vi "Panel.vi"(11 "CheckboxControlEditorPanel in":refnum<class "CheckboxControlEditorPanel.lvclass">) -> ()   [LabVIEW 2020, in "VolatusGUIControls.lvlib" / "CheckboxControlEditorPanel.lvclass"]
uses:
  CheckboxControlEditorPanel.lvclass
  C:/dev/lv20CE/relink/volatus-gui-controls/VolatusGUIEditorCore/ElementEditorPanel/ElementEditorPanel.lvclass
  C:/dev/lv20CE/relink/lv-oopanel/OOPanel/Panel/Panel.lvclass
  lv-oopanel/OOPanel/Panel/Basic UI State.ctl
  lv-autocomplete/AutoComplete/AutoComplete/AutoComplete.lvclass/AutoComplete.ctl
  CheckboxControlEditorPanel.lvclass/CheckboxControlEditorPanel.ctl
  lv-autocomplete/AutoComplete/Launch Autocomplete Handler.vi
  lv-autocomplete/AutoComplete/AutoComplete/AutoComplete.lvclass
  lv-oopanel/OOPanel/Panel/Panel.lvclass
  lv-oopanel/OOPanel/OOPanel.lvlib
  VolatusGUIEditorCore/ElementEditorPanel/ElementEditorPanel.lvclass
  VolatusGUIEditorCore/VolatusGUIEditorCore.lvlib
panel:
  in  "Top":i32
  in  "Left":i32
  in  "Height":u16
  in  "Width":u16
  in  "Label Text Color":u32(colorbox) caption="Color"
  in  "Label Visible":bool caption="Visible"
  in  "Label":string
  in  "Channel":string
  in  "True Color":u32(colorbox)
  in  "False Color":u32(colorbox)
  # "Label"
  # "False"
  # "True"
  # "Color"
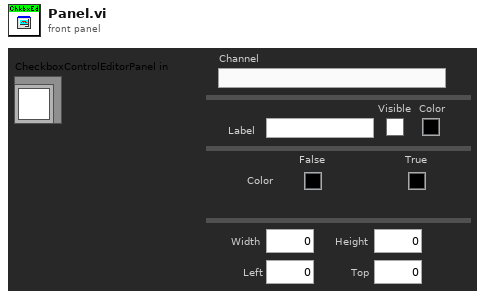
[diagram p1: front panel]
types:
  T1 = typedef "OOPanel.lvlib/Panel.lvclass/Basic UI State.ctl" = enum16{"Init", "Run", "Close"}
  T2 = typedef "VolatusGUIEditorCore.lvlib/ElementEditorPanel.lvclass/Incoming Events.ctl" = cluster{"Update Control":refnum<user-event>}
  T3 = typedef "OOPanel.lvlib/Panel.lvclass/Panel Events.ctl" = cluster{"Visbility":refnum<user-event>, "Close":refnum<user-event>}
  T4 = typedef "VolatusGUIControls.lvlib/CheckboxControlEditorPanel.lvclass/Props.ctl" = cluster{"JSON":T5, "Label":T6, "Position":T7, "Width":u16, "Height":u16, "Boolean Colors":T8}
  T5 = typedef "VolatusGUIControls.lvlib/CheckboxControlEditorPanel.lvclass/JSON Props.ctl" = cluster{"Channel":string}
  T6 = typedef "VolatusGUIEditorCore.lvlib/Label Props.ctl" = cluster{"Text":string, "Text Color":u32, "Visible":bool}
  T7 = typedef "VolatusGUIEditorCore.lvlib/Position Props.ctl" = cluster{"Left":i32, "Top":i32}
  T8 = typedef "VolatusGUIEditorCore.lvlib/Boolean Color Props.ctl" = cluster{"False":u32, "True":u32}
  T9 = typedef "OOPanel.lvlib/Visibility State.ctl" = enum16{"Idle", "Closed", "Hidden", "Visible", "Subpanel", "Hidden Subpanel"}
  T10 = cluster{"Label":string, "Label Text Color":u32, "Label Visible":bool}
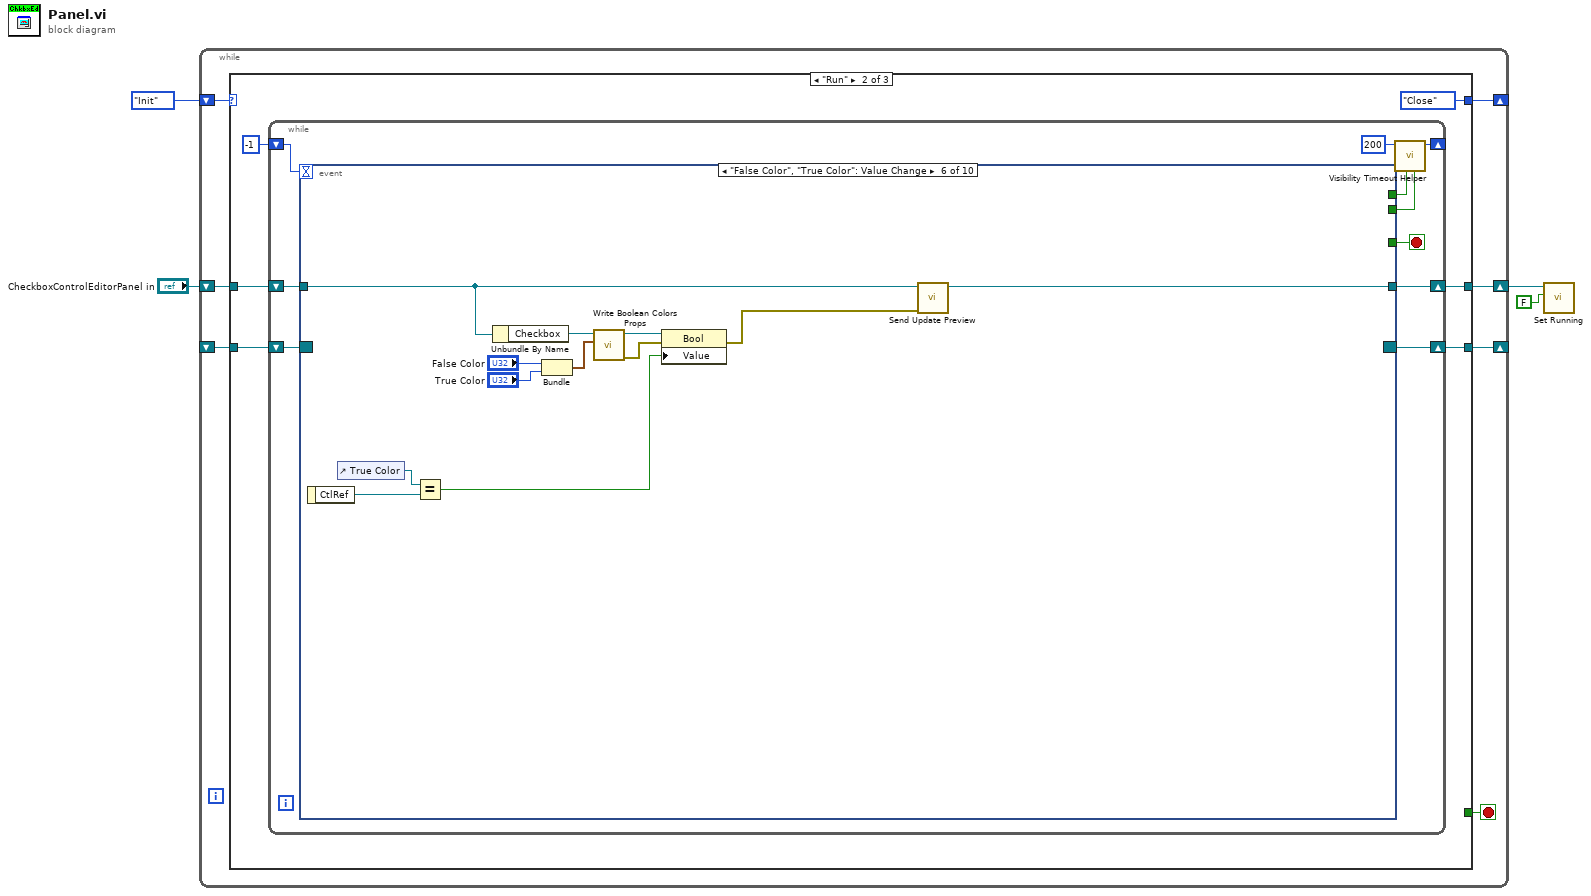
[diagram p0: block diagram]
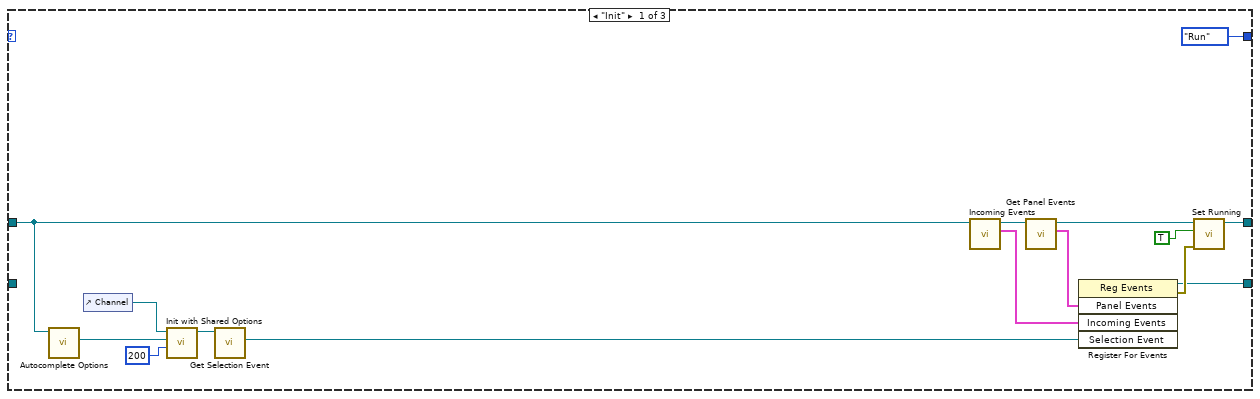
[diagram p2: hidden frame]
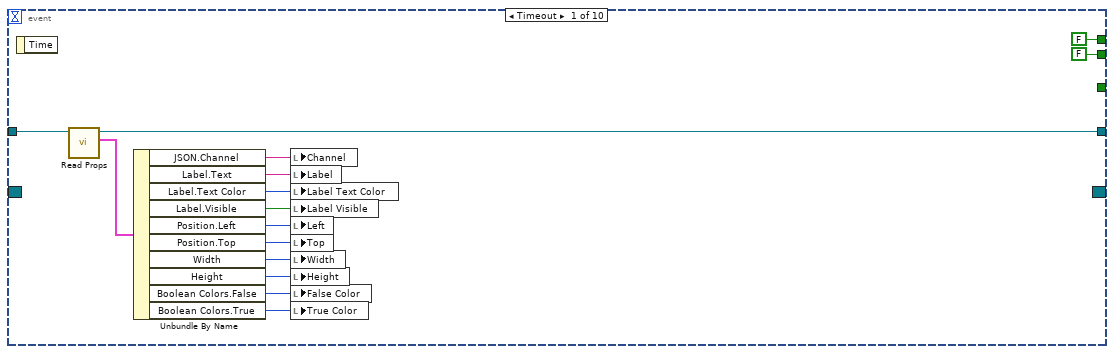
[diagram p3: hidden frame]
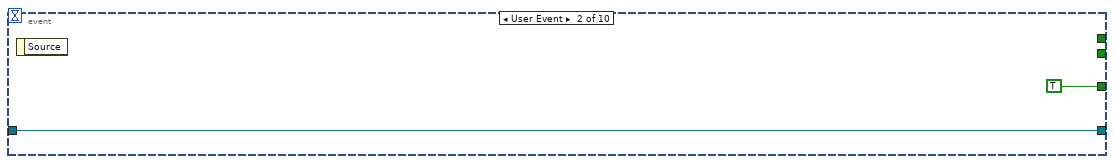
[diagram p4: hidden frame]
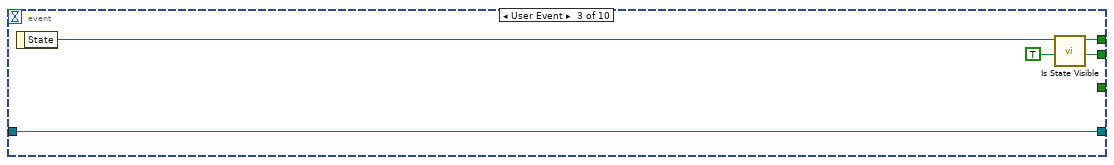
[diagram p5: hidden frame]
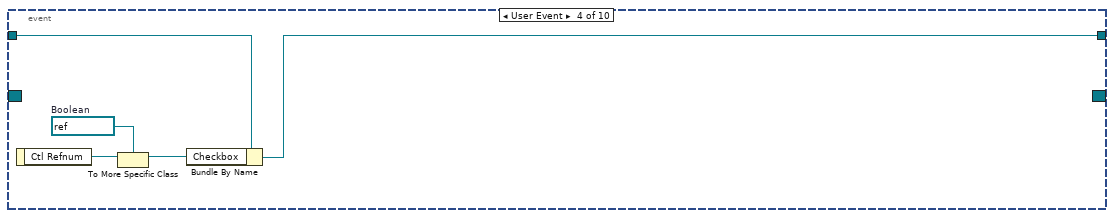
[diagram p6: hidden frame]
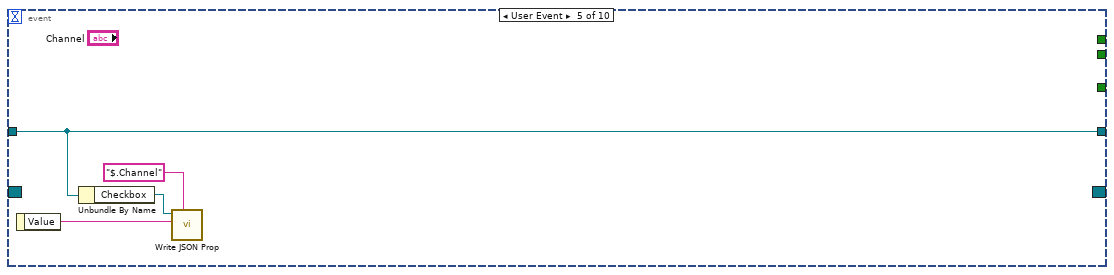
[diagram p7: hidden frame]
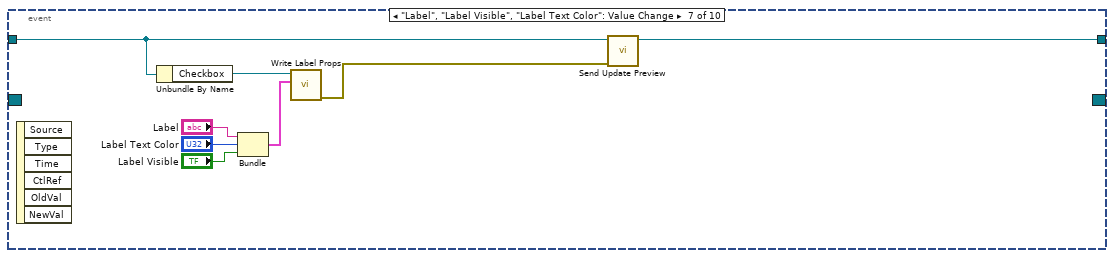
[diagram p8: hidden frame]
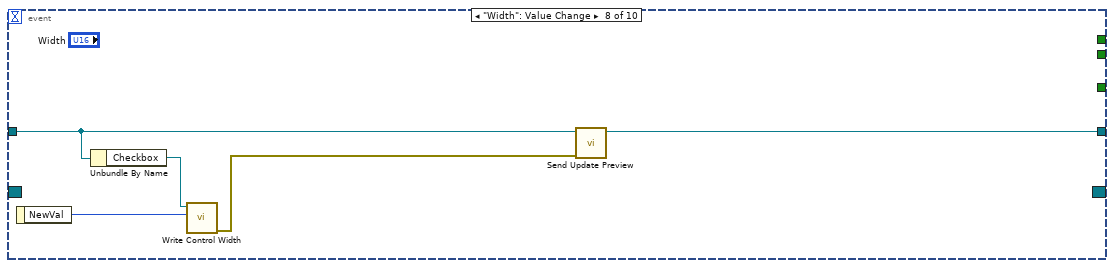
[diagram p9: hidden frame]
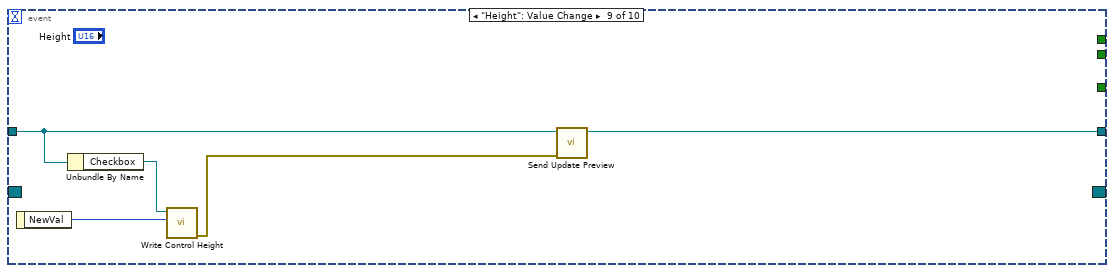
[diagram p10: hidden frame]
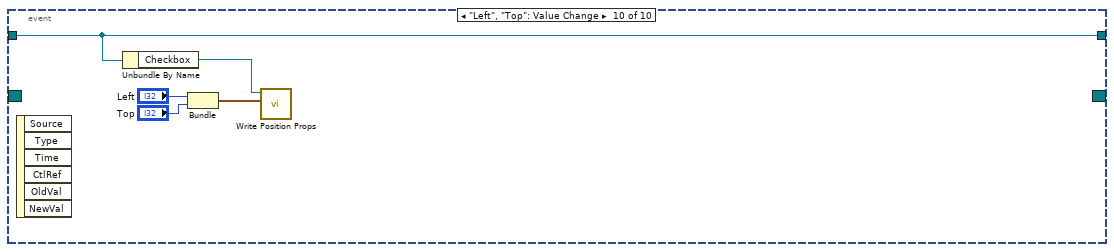
[diagram p11: hidden frame]
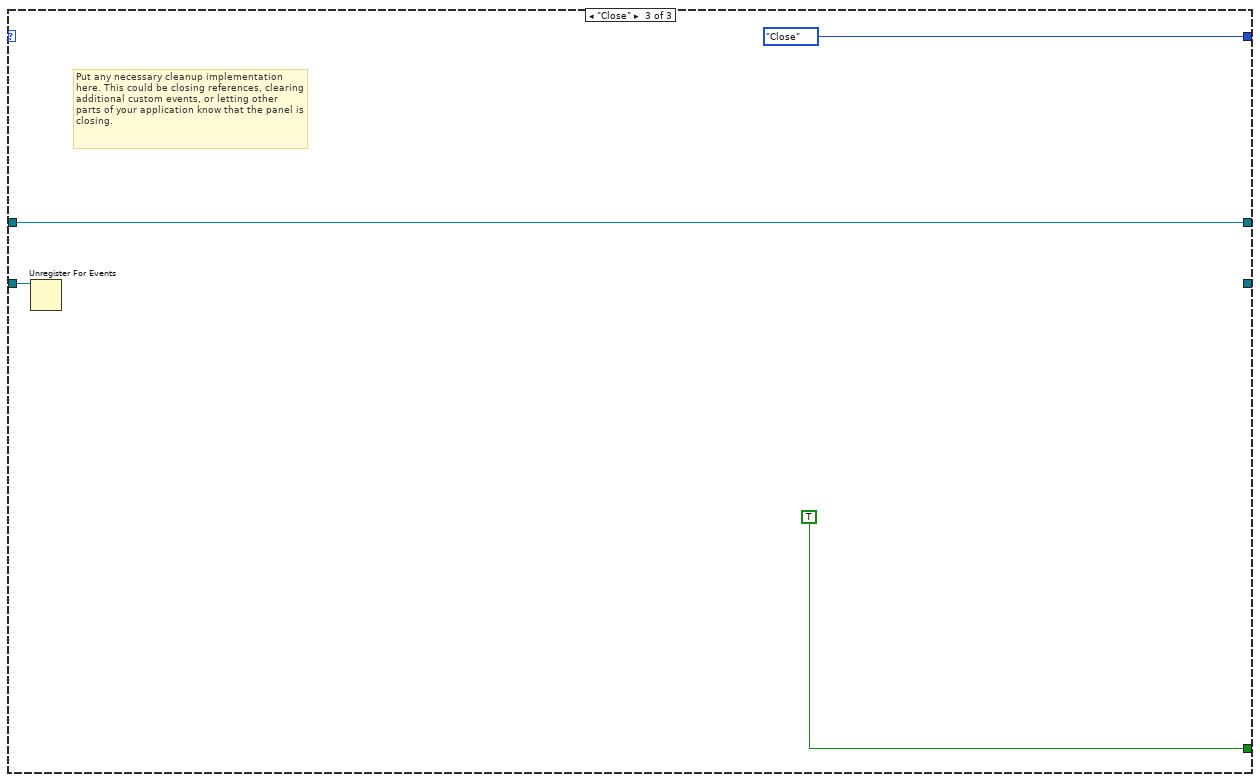
[diagram p12: hidden frame]
diagram:
  n1 = while {
    shift-right: [w10] -> _
    shift-left: _ -> [w11]
    shift-right: [w8] -> _
    shift-left: Basic_UI_State."Init" ("Basic UI State") -> [w9]
    shift-right: [w6] -> w4
    shift-left: "CheckboxControlEditorPanel in" -> [w5]
    stop <- w7 stop-if-true
    n2 = case shown="\"Run\"" w9 {
      tunnel: w11 -> [_ w32 w109]
      tunnel: [w23 w30 _] -> w10
      tunnel: [Basic_UI_State."Run" ("Basic UI State") Basic_UI_State."Close" ("Basic UI State") Basic_UI_State."Close" ("Basic UI State")] -> w8
      tunnel: [_ _ TRUE] -> w7
      tunnel: [w22 w27 w108] -> w6
      tunnel: w5 -> [w14 w28 w108]
      frame "Init" {
        n3 = call "Autocomplete Options.vi"("ElementEditorPanel in"=w14) -> ("Autocomplete Options"=w17:refnum<class "Shared Options.lvclass">)  [unwired: 10 in]
        n4 = control-ref of="Channel"() -> (w12:refnum<vi>)
        n5 = call "Init with Shared Options.vi"("Height (200)"=i16 200, "Shared Options"=w17, "Str Refnum"=w12) -> ("AutoComplete out"=w16:refnum<class "AutoComplete.lvclass">)  [unwired: 7 in, 1 out]
        n6 = call "Get Selection Event.vi"("AutoComplete in"=w16) -> ("Selection Event"=w13:refnum<user-event>)  [unwired: 9 in, 1 out]
        n7 = call "Incoming Events.vi"("ElementEditorPanel in"=w14) -> ("Incoming Events"=w18:T2, "ElementEditorPanel out"=w19:refnum<class "CheckboxControlEditorPanel.lvclass">)  [unwired: 9 in]
        n8 = call "Get Panel Events.vi"("Panel in"=w19) -> ("Panel Events"=w20:T3, "Panel out"=w21:refnum<class "CheckboxControlEditorPanel.lvclass">)  [unwired: 8 in, 1 out]
        n9 = register-events(w20, w18, w13) -> (reference out=w23:refnum<event-registration>, error out=w25:errorcluster)  [unwired: 2 in]
        n10 = call "Set Running.vi"("error in (no error)"=w25, "Running"=TRUE, "Panel in"=w21) -> ("Panel out"=w22:refnum<class "CheckboxControlEditorPanel.lvclass">)  [unwired: 7 in, 1 out]
      }
      frame "Run" {
        n11 = while {
          shift-right: [w38] -> w30
          shift-left: w32 -> [w39]
          shift-right: [w41] -> _
          shift-left: -1 ("Timeout") -> [w40]
          shift-right: [w33] -> w27
          shift-left: w28 -> [w34]
          stop <- w35 stop-if-true
          n12 = event shown="[5] \"False Color\", \"True Color\": Value Change" {
            selector: w39 -> [_ _ _ _ _ _ _ _ _ _]
            dyn-events: [_ _ _ _ _ _ _ _ _ _] -> w38
            timeout: w40 -> [_ _ _ _ _ _ _ _ _ _]
            tunnel: [FALSE _ w62 _ _ _ _ _ _ _] -> w37
            tunnel: [FALSE _ TRUE _ _ _ _ _ _ _] -> w36
            tunnel: [_ TRUE _ _ _ _ _ _ _ _] -> w35
            tunnel: w34 -> [w54 w58 w60 w68 w70 w81 w88 w97 w102 w105]
            tunnel: [w55 w58 w60 w65 w70 w79 w86 w94 w99 w105] -> w33
            event Timeout {
              n13 = event-data() -> ()  [unwired: 1 in, 1 out]
              n14 = call "Read Props.vi"("CheckboxControlEditorPanel in"=w54) -> ("Props"=w53:T4, "CheckboxControlEditorPanel out"=w55:refnum<class "CheckboxControlEditorPanel.lvclass">)  [unwired: 8 in, 1 out]
              n15 = Unbundle By Name(w53) -> ("JSON.Channel"=w52:string, "Label.Text"=w43:string, "Label.Text Color"=w51:u32, "Label.Visible"=w50:bool, "Position.Left"=w49:i32, "Position.Top"=w48:i32, "Width"=w47:u16, "Height"=w46:u16, "Boolean Colors.False"=w45:u32, "Boolean Colors.True"=w44:u32)
              n16 = local write "Channel"(w52) -> ()
              n17 = local write "Label"(w43) -> ()
              n18 = local write "Label Text Color"(w51) -> ()
              n19 = local write "Label Visible"(w50) -> ()
              n20 = local write "Left"(w49) -> ()
              n21 = local write "Top"(w48) -> ()
              n22 = local write "Width"(w47) -> ()
              n23 = local write "Height"(w46) -> ()
              n24 = local write "False Color"(w45) -> ()
              n25 = local write "True Color"(w44) -> ()
            }
            event User Event {
              n26 = event-data() -> ()  [unwired: 1 in, 1 out]
            }
            event User Event {
              n27 = event-data() -> ("State"=w63:T9)  [unwired: 1 in]
              n28 = call "Is State Visible.vi"("Visibility"=w63) -> ("Visible"=w62:bool)  [unwired: 10 in]
            }
            event User Event {
              w66 = refnum<vi> refnum  # Boolean
              n29 = event-data() -> ("Ctl Refnum"=w67:refnum<vi>)  [unwired: 1 in]
              n30 = To More Specific Class(target class=w66, reference=w67) -> (specific class reference=w64:refnum<vi>)  [unwired: 1 in, 1 out]
              n31 = Bundle By Name(cluster=w68, "Checkbox"=w64) -> (w65:refnum<class "CheckboxControlEditorPanel.lvclass">)
            }
            event User Event {
              n32 = event-data() -> ("Value"=w69:string)  [unwired: 1 in]
              n33 = Unbundle By Name(w70) -> ("Checkbox"=w72:refnum<vi>)
              n34 = call "Write JSON Prop.vi"("JSON Path"="$.Channel" ("$Path or Item Name"), "Value"=w69, "Ctl Refnum in"=w72) -> ()  [unwired: 7 in, 2 out]
            }
            event "False Color", "True Color": Value Change {
              n35 = event-data() -> ("CtlRef"=w78:refnum<vi>)  [unwired: 1 in]
              n36 = control-ref of="True Color"() -> (w77:refnum<vi>)
              n37 = Equal?(x=w77, y=w78) -> (x = y?=w74:bool)
              n38 = Unbundle By Name(w81) -> ("Checkbox"=w80:refnum<vi>)
              n39 = Bundle("False Color"="False Color", "True Color"="True Color") -> (w82:cluster{"False Color":u32, "True Color":u32})  [unwired: 1 in]
              n40 = call "Write Boolean Colors Props.vi"("Boolean Colors Props"=w82, "Control in"=w80) -> ("error out"=w75:errorcluster, "Control"=w76:refnum<vi>)  [unwired: 8 in]
              n41 = property class="Bool"(reference=w76, error in=w75, "Value"=w74) -> (error out=w73:errorcluster)  [unwired: 1 out]
              n42 = call "Send Update Preview.vi"("error in (no error)"=w73, "ElementEditorPanel in"=w81) -> ("ElementEditorPanel out"=w79:refnum<class "CheckboxControlEditorPanel.lvclass">)  [unwired: 8 in, 1 out]
            }
            event "Label", "Label Visible", "Label Text Color": Value Change {
              n43 = event-data() -> ()  [unwired: 1 in, 6 out]
              n44 = Unbundle By Name(w88) -> ("Checkbox"=w87:refnum<vi>)
              n45 = Bundle("Label"="Label", "Label Text Color"="Label Text Color", "Label Visible"="Label Visible") -> (w89:T10)  [unwired: 1 in]
              n46 = call "Write Label Props.vi"("Label Props"=w89, "Ctl Refnum in"=w87) -> ("error out"=w85:errorcluster)  [unwired: 8 in, 1 out]
              n47 = call "Send Update Preview.vi"("error in (no error)"=w85, "ElementEditorPanel in"=w88) -> ("ElementEditorPanel out"=w86:refnum<class "CheckboxControlEditorPanel.lvclass">)  [unwired: 8 in, 1 out]
            }
            event "Width": Value Change {
              n48 = event-data() -> ("NewVal"=w95:u16)  [unwired: 1 in]
              n49 = Unbundle By Name(w97) -> ("Checkbox"=w96:refnum<vi>)
              n50 = call "Write Control Width.vi"("Width"=w95, "Control in"=w96) -> ("error out"=w93:errorcluster)  [unwired: 8 in, 1 out]
              n51 = call "Send Update Preview.vi"("error in (no error)"=w93, "ElementEditorPanel in"=w97) -> ("ElementEditorPanel out"=w94:refnum<class "CheckboxControlEditorPanel.lvclass">)  [unwired: 8 in, 1 out]
            }
            event "Height": Value Change {
              n52 = event-data() -> ("NewVal"=w100:u16)  [unwired: 1 in]
              n53 = Unbundle By Name(w102) -> ("Checkbox"=w101:refnum<vi>)
              n54 = call "Write Control Height.vi"("Height"=w100, "Control in"=w101) -> ("error out"=w98:errorcluster)  [unwired: 8 in, 1 out]
              n55 = call "Send Update Preview.vi"("error in (no error)"=w98, "ElementEditorPanel in"=w102) -> ("ElementEditorPanel out"=w99:refnum<class "CheckboxControlEditorPanel.lvclass">)  [unwired: 8 in, 1 out]
            }
            event "Left", "Top": Value Change {
              n56 = event-data() -> ()  [unwired: 1 in, 6 out]
              n57 = Unbundle By Name(w105) -> ("Checkbox"=w104:refnum<vi>)
              n58 = Bundle("Left"="Left", "Top"="Top") -> (w103:cluster{"Left":i32, "Top":i32})  [unwired: 1 in]
              n59 = call "Write Position Props.vi"("Position Props"=w103, "Ctl Refnum in"=w104) -> ()  [unwired: 8 in, 2 out]
            }
          }
          n60 = call "Visibility Timeout Helper.vi"("Update?"=w36, "Use Timeout?"=w37, "Visible Timeout mS"=200) -> ("Timeout"=w41:i32)  [unwired: 8 in]
        }
      }
      frame "Close" {
        # "Put any necessary cleanup implementation here. This could be closing references, clearing additional custom events, or letting other parts of your application know that the panel is closing."
        n61 = Unregister For Events(event registration refnum=w109) -> ()  [unwired: 1 in, 1 out]
      }
    }
  }
  n62 = call "Set Running.vi"("Running"=FALSE, "Panel in"=w4) -> ()  [unwired: 8 in, 2 out]
